vi "ARRAY VARIABLES.vi"(7 "TIMESTAMP":dbl[](array[numeric])=[1464082271000.0, 1464082271000.0, 1464082271000.0, 1464082271000.0], 9 "VELOCIDAD":dbl[](array[numeric])=[10.0, 10.0, 10.0, 10.0], 10 "TAGS":string[][](array[string])=[["taginiLinea6", "tagfinLinea6"], ["taginiLinea6", "tagfinLinea6"], ["taginiLinea6", "tagfinLinea6"], ["taginiLinea6", "tagfinLinea6"]], 11 "TEMPER":dbl[](array[numeric])=[40.0, 40.0, 40.0, 40.0]) -> (0 "ARRAY TAGS":string[](array[string]), 1 "ARRAY TIMESTAMP":dbl, 2 "ARRAY VELOCIDAD":dbl, 3 "TEMPERATURA":dbl)   [LabVIEW 2015]
panel:
  out "size(s)":i32
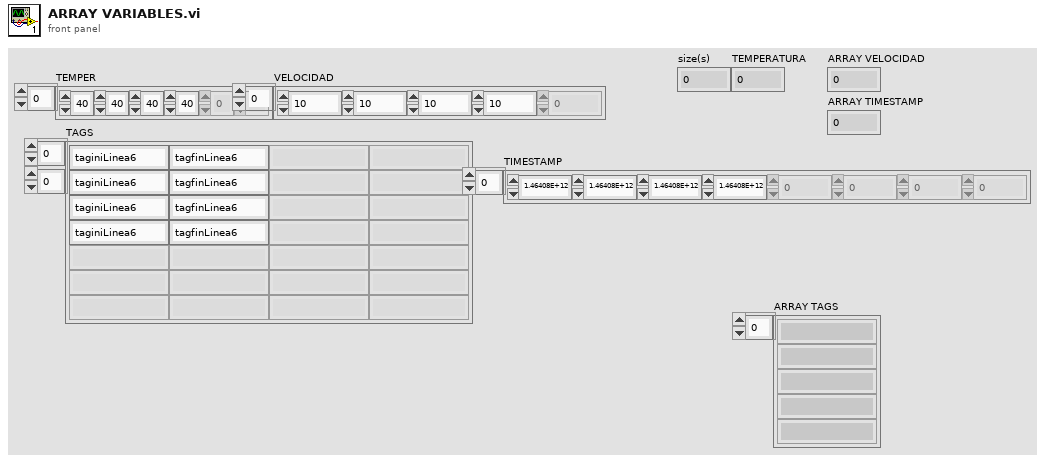
[diagram p1: front panel]
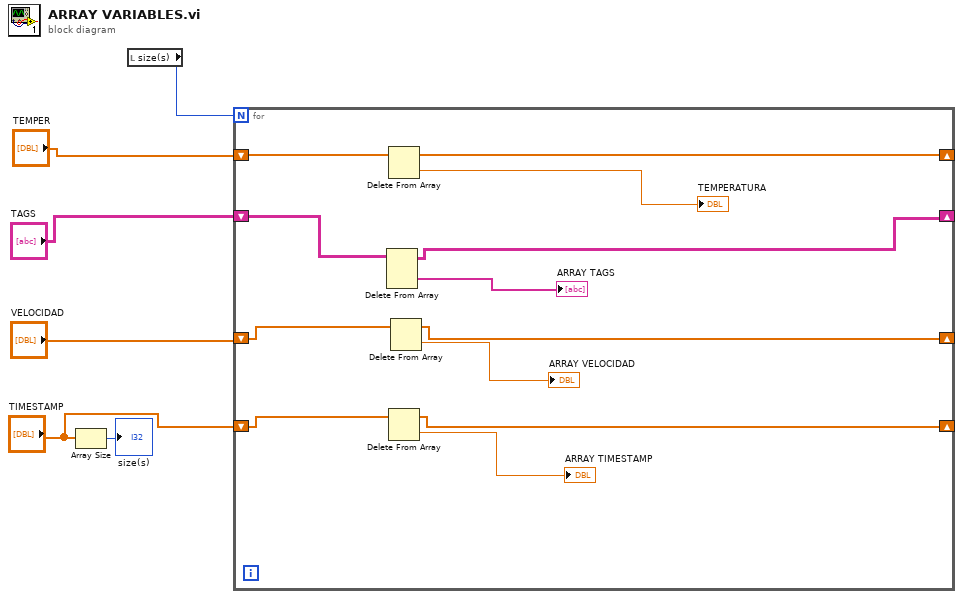
[diagram p0: block diagram]
diagram:
  n1 = Array Size(array="TIMESTAMP") -> (size(s)=→"size(s)":i32)
  n2 = local read "size(s)"() -> (w5:i32)
  n3 = for {
    N: w5 -> [_]
    shift-right: [w17] -> _
    shift-left: "TEMPER" -> [w18]
    shift-right: [w14] -> _
    shift-left: "TAGS" -> [w15]
    shift-right: [w12] -> _
    shift-left: "VELOCIDAD" -> [w13]
    shift-right: [w10] -> _
    shift-left: "TIMESTAMP" -> [w11]
    n4 = Delete From Array(array=w15) -> (deleted portion=→"ARRAY TAGS":string[], array with subset deleted=w14:string[][])  [unwired: 3 in]
    n5 = Delete From Array(array=w18) -> (deleted portion=→"TEMPERATURA":dbl, array with subset deleted=w17:dbl[])  [unwired: 2 in]
    n6 = Delete From Array(array=w11) -> (deleted portion=→"ARRAY TIMESTAMP":dbl, array with subset deleted=w10:dbl[])  [unwired: 2 in]
    n7 = Delete From Array(array=w13) -> (deleted portion=→"ARRAY VELOCIDAD":dbl, array with subset deleted=w12:dbl[])  [unwired: 2 in]
  }
